vi "LSM PreFlight Z-Stack.vi"(8 "error in (no error)":errorcluster, 11 "Start":dbl) -> (0 "error out":errorcluster, 2 "ID out":i32, 3 "pDataBuffer":u16[](array[numeric]))   [LabVIEW 2020]
uses:
  Instruments/Physik Instrumente/SDK/GCS_LabVIEW_digital/Low Level/Communication.llb/Global1.vi
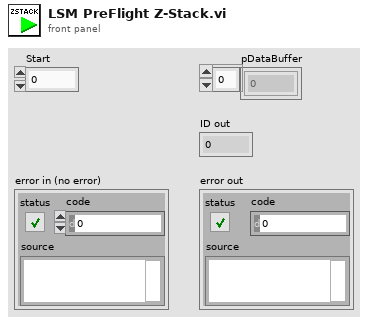
[diagram p1: front panel]
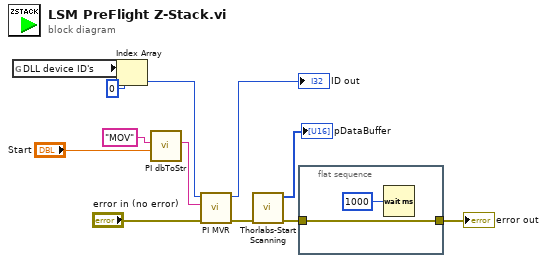
[diagram p0: block diagram]
diagram:
  n1 = global read "Global1.vi" "DLL device ID's"() -> (w6:i32[])
  n2 = Index Array(array=w6, index=0) -> (element=w3:i32)
  n3 = call "PI dbToStr.vi"("Start"="Start", "String in"="MOV") -> ("String out"=w2:string)  [unwired: 9 in]
  n4 = call "PI MVR.vi"("error in (no error)"="error in (no error)", "String"=w2, "PI ID in"=w3) -> ("error out"=w8:errorcluster, "PI ID out"=→"ID out":i32)  [unwired: 6 in, 1 out]
  n5 = call "Thorlabs-Start Scanning.vi"("error in (no error)"=w8) -> ("error out"=w11:errorcluster, "pDataBuffer"=→"pDataBuffer":u16[])  [unwired: 9 in]
  n6 = flat-sequence {
    tunnel: [w14] -> w10
    tunnel: w11 -> [w14]
    frame #0 {
      n7 = Wait (ms)(milliseconds to wait=u32 1000) -> ()  [unwired: 1 out]
    }
  }
  "error out" <- w10
